vi "NTLogger.vi"(10 "error in (no error)":errorcluster) -> ()   [LabVIEW 2015]
uses:
  <vilib>/Rock Robotics/WPI/DriverStation/WPI_DriverStationRobotMode2.ctl
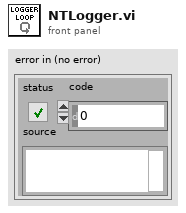
[diagram p1: front panel]
types:
  T1 = enum16{"open", "replace", "create", "open or create", "replace or create", "replace or create with confirmation"}
  T2 = typedef "WPI_DriverStationRobotMode2.ctl" = enum16{"Autonomous Disabled", "Autonomous Enabled", "Teleop Disabled", "Teleop Enabled", "Disconnected", "Finish", "Test Disabled", "Test Enabled", "Emergency Stopped"}
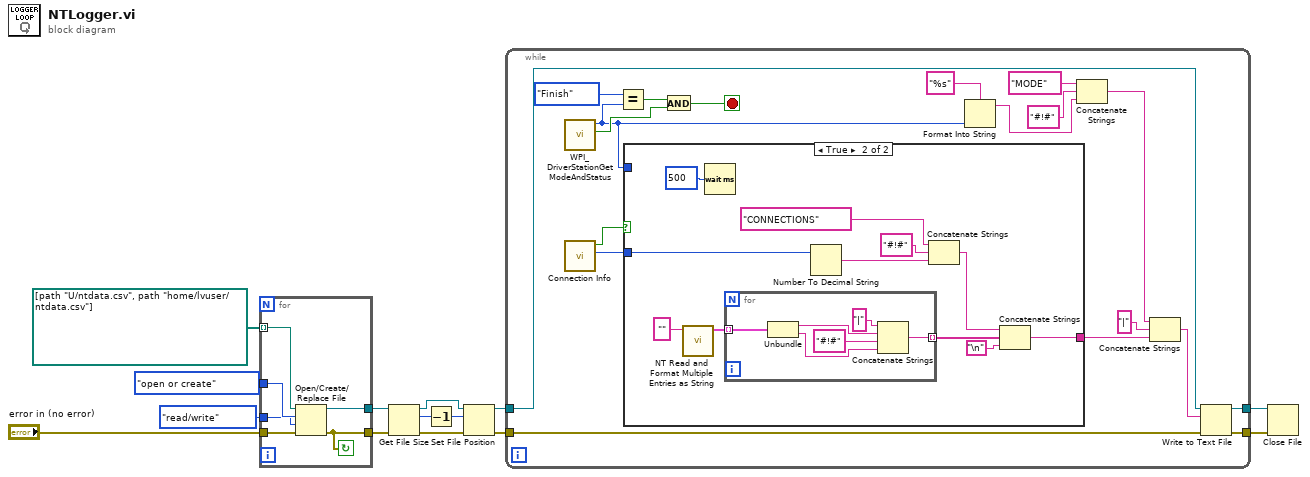
[diagram p0: block diagram]
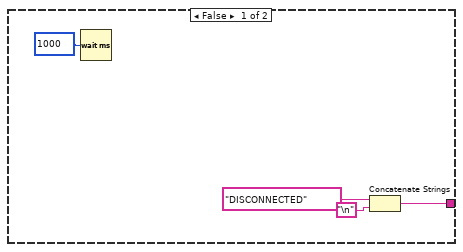
[diagram p2: hidden frame]
diagram:
  n1 = for {
    tunnel: [w20] -> w8
    tunnel: T1."open or create" ("operation (0:open)") -> [w18]
    tunnel: enum16{"read/write", "read-only", "write-only"}."read/write" ("access (0:read/write)") -> [w17]
    tunnel: "error in (no error)" -> [w19]
    tunnel: [w15] -> w7
    tunnel: path[] [path "U:/ntdata.csv", path "/home/lvuser/ntdata.csv"] -> [w16] mode=indexing
    stop <- w15 continue-if-true
    n2 = Open/Create/Replace File(file path (use dialog)=w16, error in=w19, operation (0:open)=w18, access (0:read/write)=w17) -> (refnum out=w20:refnum<file>, error out=w15:errorcluster)  [unwired: 2 in, 1 out]
  }
  n3 = Get File Size(file=w8, error in=w7) -> (refnum out=w4:refnum<file>, size (in bytes)=w5:i64, 0:w6:errorcluster)
  n4 = Decrement(x=w5) -> (x-1=w1:i64)
  n5 = Set File Position(offset (in bytes) (0)=w1, refnum=w4, error in=w6) -> (refnum out=w3:refnum<file>, error out=w2:errorcluster)  [unwired: 1 in]
  n6 = while {
    tunnel: w3 -> [w36]
    tunnel: w2 -> [w37]
    tunnel: [w35] -> w11
    tunnel: [w34] -> w10
    stop <- w30 stop-if-true
    n7 = call <vilib>:"WPI_DriverStationGetModeAndStatus.vi"() -> ("FMS Attached"=w32:bool, "Robot Mode"=w25:T2)  [unwired: 10 in]
    n8 = call <vilib>:"Connection Info.vi"() -> ("Connection Count"=w38:i32, "Connected"=w39:bool)  [unwired: 10 in]
    n9 = Equal?(x=WPI_DriverStationRobotMode2."Finish" ("y"), y=w25) -> (x = y?=w31:bool)
    n10 = case shown="True" w39 {
      tunnel: w38 -> [_ w51]
      tunnel: [w41 w50] -> w23
      tunnel: w25 -> [_ _]
      frame False {
        n11 = Wait (ms)(milliseconds to wait=u32 1000) -> ()  [unwired: 1 out]
        n12 = Concatenate Strings("DISCONNECTED" ("string"), "\n") -> (w41:string)
      }
      frame True {
        n13 = call <vilib>:"NT Read and Format Multiple Entries as String.vi"("Name Pattern"="") -> ("Formatted Strings"=w53:cluster{"Name":string, "Value":string}[])  [unwired: 9 in, 1 out]
        n14 = Wait (ms)(milliseconds to wait=u32 500) -> ()  [unwired: 1 out]
        n15 = for {
          tunnel: w53 -> [w60] mode=indexing
          tunnel: [w56] -> w46 mode=indexing
          n16 = Unbundle(w60) -> ("Name"=w59:string, "Value"=w58:string)
          n17 = Concatenate Strings("|" ("string"), w59, "#!#" ("string"), w58) -> (w56:string)
        }
        n18 = Number To Decimal String(number=w51) -> (decimal integer string=w48:string)  [unwired: 1 in]
        n19 = Concatenate Strings("CONNECTIONS" ("string"), "#!#" ("string"), w48) -> (w49:string)
        n20 = Concatenate Strings(w49, w46, "\n") -> (w50:string)
      }
    }
    n21 = And(x=w31, y=w32) -> (x .and. y?=w30:bool)
    n22 = Format Into String(format string="%s", w25) -> (resulting string=w28:string)  [unwired: 2 in, 1 out]
    n23 = Concatenate Strings("MODE" ("string"), "#!#" ("string"), w28) -> (w21:string)
    n24 = Concatenate Strings(w21, "|" ("string"), w23) -> (w22:string)
    n25 = Write to Text File(file (use dialog)=w36, text=w22, error in=w37) -> (refnum out=w35:refnum<file>, error out=w34:errorcluster)  [unwired: 1 in, 1 out]
  }
  n26 = Close File(refnum=w11, error in=w10) -> ()  [unwired: 2 out]
